vi "slice_osq.vi"(9 "VAR":string, 11 "SEQs in":T1[](array[typedef])) -> (2 "VALS":string[](array[string]), 3 "SEQs out":T1[](array[typedef]))   [LabVIEW 2013]
uses:
  Line.ctl
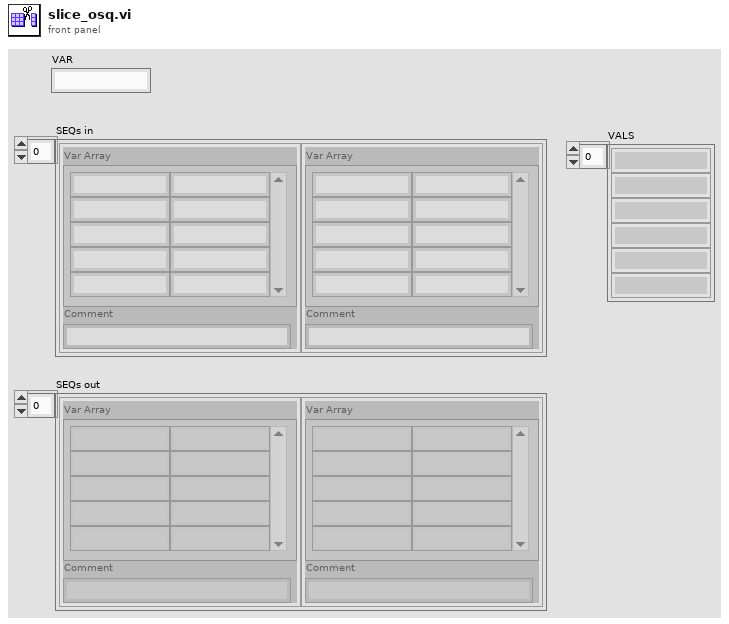
[diagram p1: front panel]
types:
  T1 = typedef "Line.ctl" = cluster{"Var Array":string[][], "Comment":string}
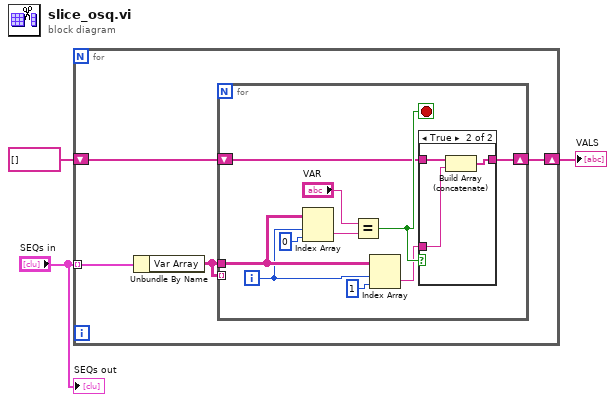
[diagram p0: block diagram]
diagram:
  n1 = for {
    tunnel: "SEQs in" -> [w7] mode=indexing
    shift-right: [w6] -> w1
    shift-left: string[] [] -> [w5]
    n2 = Unbundle By Name(w7) -> ("Var Array"=w4:string[][])
    n3 = for {
      tunnel: w4 -> [w17]
      shift-right: [w12] -> w6
      shift-left: w5 -> [w11]
      tunnel: w4 -> [_] mode=indexing
      i -> [w10]
      stop <- w14 stop-if-true
      n4 = Index Array(array=w17, index (row)=w10, index (col)=0 ("disabled index (col)")) -> (element=w16:string)
      n5 = Equal?(x="VAR", y=w16) -> (x = y?=w14:bool)
      n6 = Index Array(array=w17, index (row)=w10, index (col)=1 ("disabled index (col)")) -> (element=w13:string)
      n7 = case shown="True" w14 {
        tunnel: w13 -> [_ w21]
        tunnel: [w18 w20] -> w12
        tunnel: w11 -> [w18 w19]
        frame False {
        }
        frame True {
          n8 = Build Array (concatenate)(w19, w21) -> (w20:string[])
        }
      }
    }
  }
  "VALS" <- w1
  "SEQs out" <- "SEQs in"
